vi "Sort 2D String Array - Pre-process.vi"(0 "Array to Sort In":string[][](array[string]), 4 "Input Array Contains Header Row? (T)":T1=TRUE) -> (14 "Array to Sort Out":string[][](array[string]))   [LabVIEW 2010, in "xijk_select_best_filter.lvlib"]
doc: "Sort 2D String Array - Pre-process.vi\n\n<B>Description:</B>\n\nThis VI processes the strings in the Array to Sort In input into strings that will sort properly using the Sort 1D Array function.\n\n<B>Usage:</B>\n\nWire all required inputs.\n\n<B>Inputs:</B>\n\nArray to Sort In\n- This is the input array of strings that will be sorted.\n\nInput Array Contains Header Row? (T)\n- This input indicates if the input array contains a header row.\n\n<B>Outputs:</B>\n\nArray to Sort Out\n- This is the input array of strings processed into strings that will sort properly using the Sort 1D Array function.\n\n<B>Developed by:</B>\n\nMark Ridgley\nmark.ridgley@logicpd.com"
uses:
  xijk_select_best_filter.lvlib
  _TypeDefs/TYPE - Input Array Contains Header Row.ctl
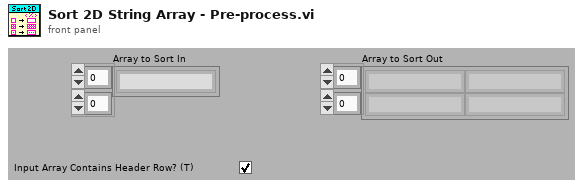
[diagram p1: front panel]
types:
  T1 = typedef "xijk_select_best_filter.lvlib/TYPE - Input Array Contains Header Row.ctl" = bool
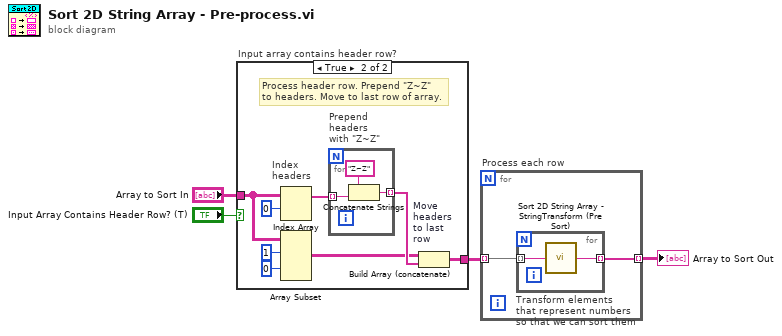
[diagram p0: block diagram]
diagram:
  n1 = case "Input array contains header row?" shown="True" "Input Array Contains Header Row? (T)" {
    tunnel: [w5 w13] -> w3
    tunnel: "Array to Sort In" -> [w5 w8]
    frame False {
      # "No header row."
    }
    frame True {
      # "Process header row. Prepend \"Z~Z\"\nto headers. Move to last row of array."
      # "Index\nheaders"
      n2 = Index Array(array=w8, index (row)=0 ("Index")) -> (element=w10:string[])  [unwired: 1 in]
      n3 = Array Subset(array=w8, index (row)=1 ("Array Index"), index (col)=0 ("Array Index")) -> (w9:string[][])  [unwired: 2 in]
      n4 = for "Prepend\nheaders\nwith \"Z~Z\"" {
        tunnel: w10 -> [w16] mode=indexing
        tunnel: [w15] -> w12 mode=indexing
        n5 = Concatenate Strings("Z~Z" ("Substring"), w16) -> (w15:string)
      }
      n6 = Build Array (concatenate) "Move\nheaders\nto last\nrow"(w9, w12) -> (w13:string[][])
    }
  }
  n7 = for "Process each row" {
    tunnel: w3 -> [w18] mode=indexing
    tunnel: [w17] -> w4 mode=indexing
    n8 = for "Transform elements\nthat represent numbers\nso that we can sort them" {
      tunnel: w18 -> [w20] mode=indexing
      tunnel: [w19] -> w17 mode=indexing
      n9 = call "Sort 2D String Array - StringTransform (Pre Sort).vi"("Input String (\" \")"=w20) -> ("Output String (\" \")"=w19:string)  [unwired: 14 out]
    }
  }
  "Array to Sort Out" <- w4
